vi "Scratch.vi"() -> ()   [LabVIEW 2019]
uses:
  CEPM.lvlib
panel:
  out "Install Command":string
  out "Preview":string
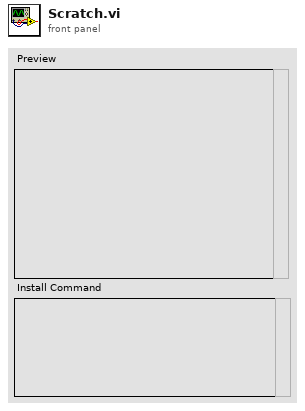
[diagram p1: front panel]
types:
  T1 = typedef "CEPM.lvlib/SystemSnapshot.ctl" = cluster{"FeedURLs":string[], "Packages":cluster{"Package":string, "Version":string}[]}
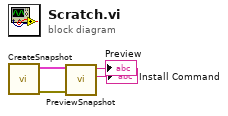
[diagram p0: block diagram]
diagram:
  n1 = call "CreateSnapshot.vi"() -> ("Error Out"=w4:errorcluster, "SystemSnapshot"=w3:T1)  [unwired: 10 in]
  n2 = call "PreviewSnapshot.vi"("Error In"=w4, "SystemSnapshot"=w3) -> ("Install Command"=→"Install Command":string, "Preview"=→"Preview":string)  [unwired: 7 in, 1 out]
